vi "SV File parser.vi"(8 "error in (no error)":errorcluster, 11 "uService ID":string="Handler") -> (0 "error out":errorcluster, 2 "Needs to Deploy":bool, 3 "SV to subscribe to":string[](array[string]))   [LabVIEW 2020, in "TALOS.lvlib" / "Father of all uServices.lvlib" / "Father of all uServices.lvclass"]
uses:
  Father of all uServices.lvclass
  25e2abe1-13bc-4007-a0e7-4f62fdb5805f.vi
  7717fe8b-e86f-413e-9362-00f50aa80320.vi
  Support VIs/Global Memory.vi
  <vilib>/Comparison/Equal/Equal Functor/Equal Functor.lvclass
  Father of all uServices.lvclass/Father of all uServices.ctl
  TALOS.lvlib
panel:
  out "data":string[][](array[string])
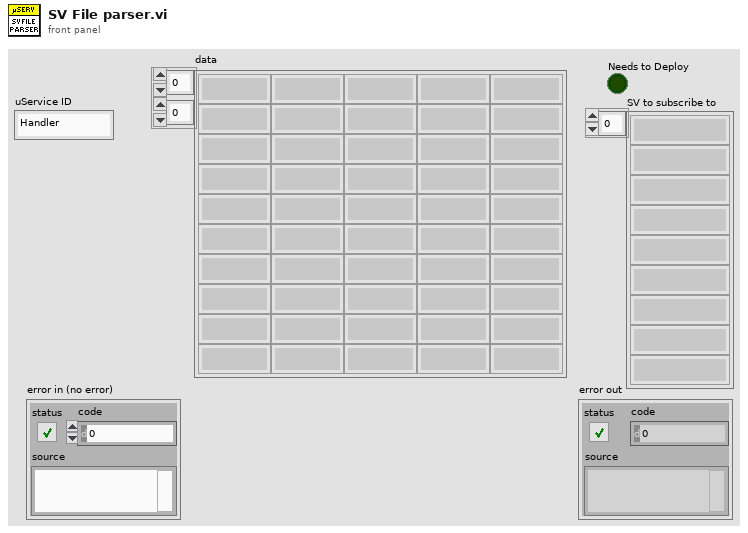
[diagram p1: front panel]
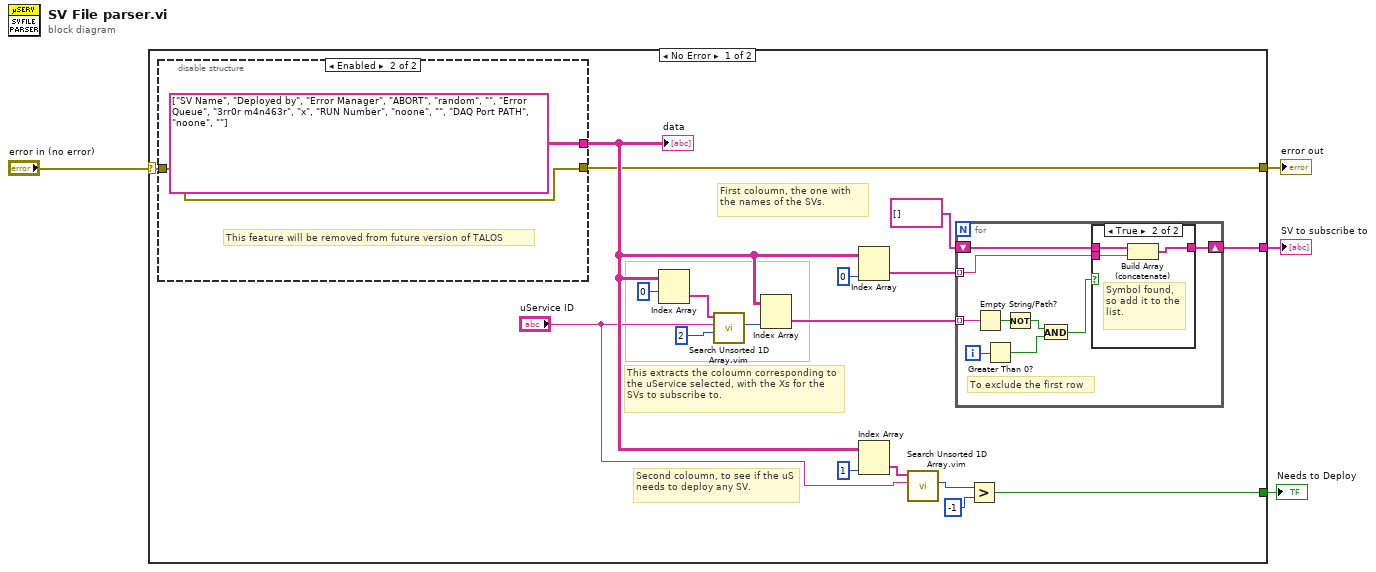
[diagram p0: block diagram]
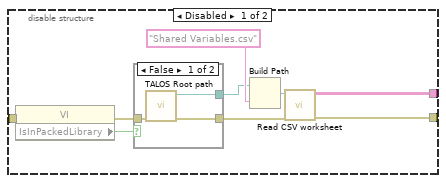
[diagram p2: hidden frame]
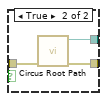
[diagram p3: hidden frame]
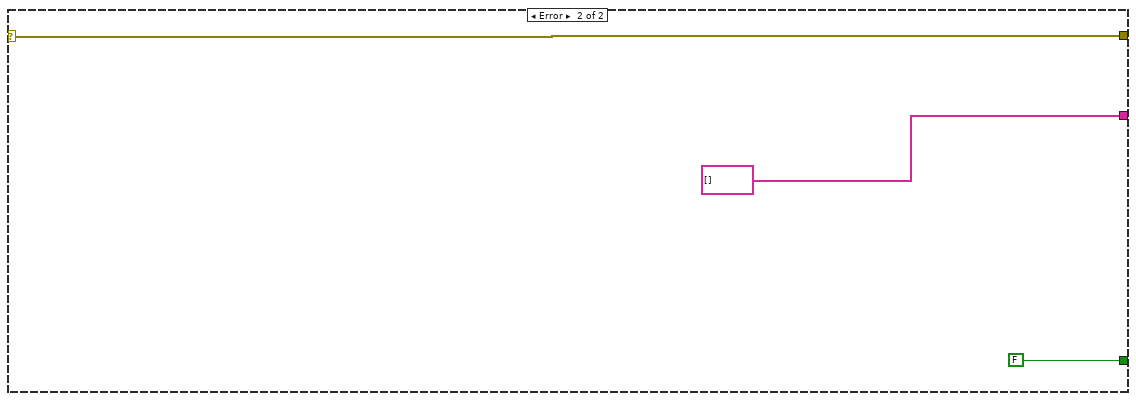
[diagram p5: hidden frame]
diagram:
  n1 = case shown="No Error" "error in (no error)" {
    selector: "error in (no error)" -> [w21 w55]
    tunnel: [w22 string[] []] -> w4
    tunnel: [w18 w55] -> w2
    tunnel: [w19 FALSE] -> w1
    frame No Error {
      # "Second coloumn, to see if the uS needs to deploy any SV."
      # "First coloumn, the one with the names of the SVs."
      # "This extracts the coloumn corresponding to the uService selected, with the Xs for the SVs to subscribe to."
      n2 = disable-structure shown="Enabled" {
        disable-tunnel: w21 -> [w31 w38]
        disable-tunnel: [w24 string[][] [["SV Name", "Deployed by", "Error Manager"], ["ABORT", "random", ""], ["Error Queue", "3rr0r m4n463r", "x"], ["RUN Number", "noone", ""], ["DAQ Port PATH", "noone", ""]]] -> w20
        disable-tunnel: [w23 w38] -> w18
        frame Disabled {
          n3 = property class="VI"(error in=w31) -> (error out=w30:errorcluster, "IsInPackedLibrary"=w29:bool)  [unwired: 1 in, 1 out]
          n4 = case shown="False" w29 {
            tunnel: [w32 w36] -> w26
            tunnel: w30 -> [w34 w37]
            tunnel: [w33 w35] -> w27
            frame False {
              n5 = call "TALOS Root path.vi"("error in (no error)"=w34) -> ("error out"=w32:errorcluster, "TALOS Root Path"=w33:path)  [unwired: 9 in]
            }
            frame True {
              n6 = call "Circus Root Path.vi"("error in (no error)"=w37) -> ("error out"=w36:errorcluster, "Circus Root Path"=w35:path)  [unwired: 9 in]
            }
          }
          n7 = Build Path(base path=w27, name or relative path="Shared Variables.csv") -> (appended path=w25:path)
          n8 = call "Read CSV worksheet.vi"("error in (no error)"=w26, "appended path"=w25) -> ("error out"=w23:errorcluster, "Sheet"=w24:string[][])  [unwired: 8 in]
        }
        frame Enabled {
          # "This feature will be removed from future version of TALOS"
        }
      }
      "data" <- w20
      n9 = Index Array(array=w20, index (row)=0) -> (element=w16:string[])  [unwired: 1 in]
      n10 = call "Search Unsorted 1D Array.vim"("start index (0)"=2, "element"="uService ID", "unsorted 1D array"=w16) -> ("index of element"=w15:i32)  [unwired: 8 in]
      n11 = Index Array(array=w20, index (col)=w15) -> (element=w11:string[])  [unwired: 1 in]
      n12 = Index Array(array=w20, index (col)=0 ("disabled index (col)")) -> (element=w12:string[])  [unwired: 1 in]
      n13 = Index Array(array=w20, index (col)=1 ("disabled index (col)")) -> (element=w8:string[])  [unwired: 1 in]
      n14 = call "Search Unsorted 1D Array.vim"("element"="uService ID", "unsorted 1D array"=w8) -> ("index of element"=w6:i32)  [unwired: 9 in]
      n15 = for {
        tunnel: w12 -> [w41] mode=indexing
        tunnel: w11 -> [w47] mode=indexing
        shift-right: [w42] -> w22
        shift-left: string[] [] -> [w43]
        i -> [w48]
        # "To exclude the first row"
        n16 = Empty String/Path?(string/path=w47) -> (empty?=w46:bool)
        n17 = Greater Than 0?(x=w48) -> (x > 0?=w45:bool)
        n18 = Not(x=w46) -> (.not. x?=w44:bool)
        n19 = And(x=w44, y=w45) -> (x .and. y?=w40:bool)
        n20 = case shown="True" w40 {
          tunnel: w43 -> [w49 w52]
          tunnel: [w49 w51] -> w42
          tunnel: w41 -> [_ w50]
          frame False {
            # "No X, so don't add it to the list."
          }
          frame True {
            # "Symbol found, so add it to the list."
            n21 = Build Array (concatenate)(w52, w50) -> (w51:string[])
          }
        }
      }
      n22 = Greater?(x=w6, y=-1) -> (0:w19:bool)
    }
    frame Error {
    }
  }
  "SV to subscribe to" <- w4
  "error out" <- w2
  "Needs to Deploy" <- w1
